vi "Turret_roller_module.vi"(0 "Reset":bool, 1 "Enable":bool, 2 "Ball Detected":bool, 3 "Ball too far":bool, 4 "Ball not far enough":bool, 5 "Lower Conveyor has Ball":bool, 6 "Shoot":bool) -> (14 "Turret Roller State":T1, 15 "T Roller Motor":dbl, 17 "Acquired Ball":bool, 18 "Accepting Balls":bool, 19 "Shot Ball":bool)   [LabVIEW 2012]
doc: "State machine for the roller buffer mounted on the turret between the tower conveyor and the flywheel."
uses:
  T_Roller module state.ctl
panel:
  in  "Shooting Timeout":u32=1000
  in  "Fast Speed":dbl=1.0
  in  "Slow Speed":dbl=0.3
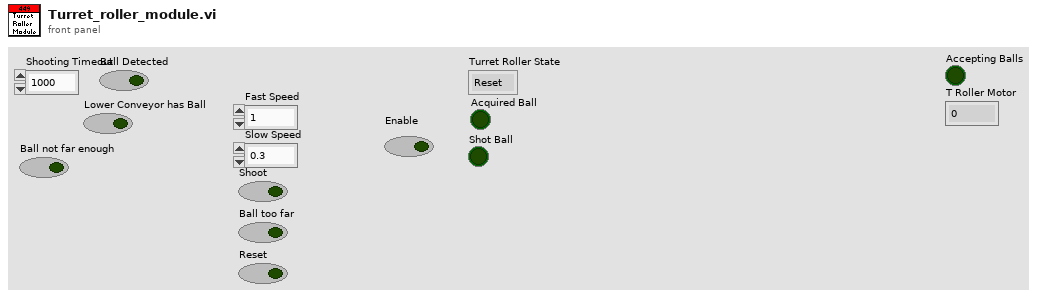
[diagram p1: front panel]
types:
  T1 = typedef "T_Roller module state.ctl" = enum16{"Reset", "Disabled", "Waiting for Ball", "Holding", "Ball not far enough", "Ball too far", "Firing"}
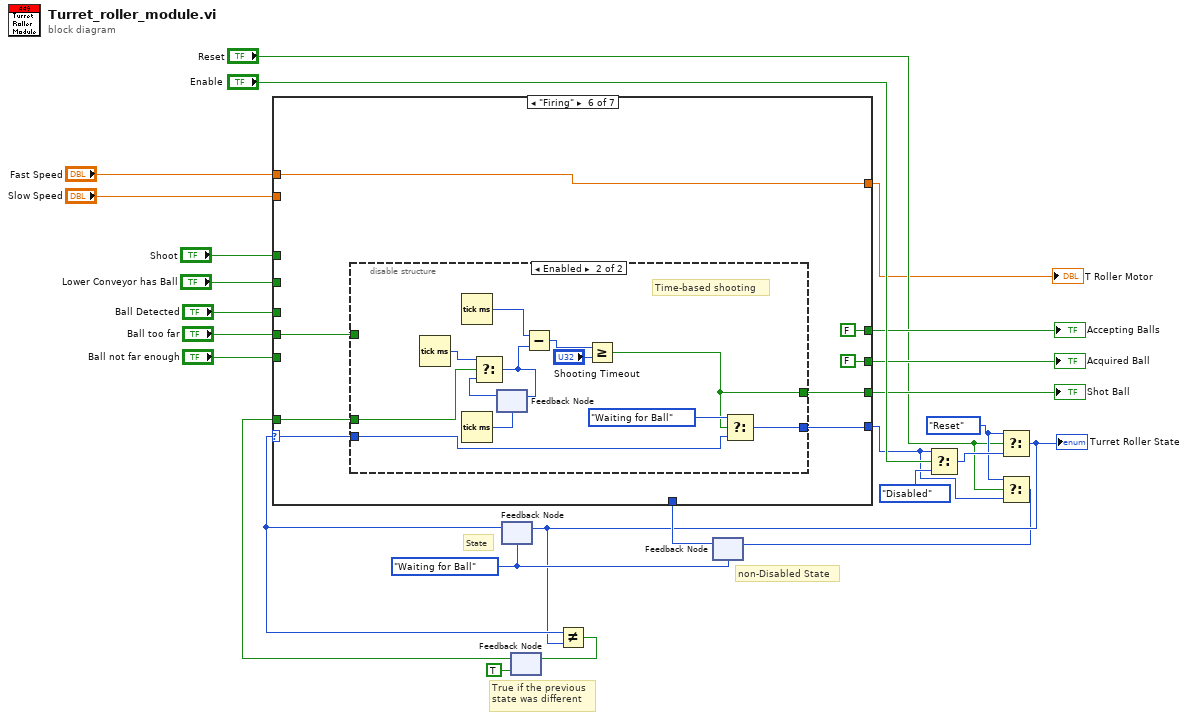
[diagram p0: block diagram]
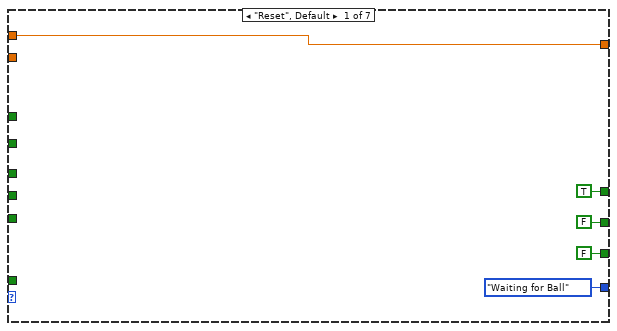
[diagram p2: hidden frame]
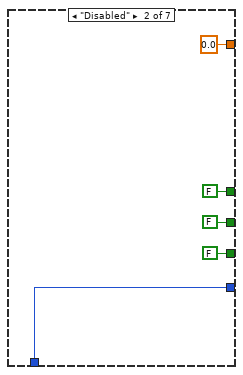
[diagram p3: hidden frame]
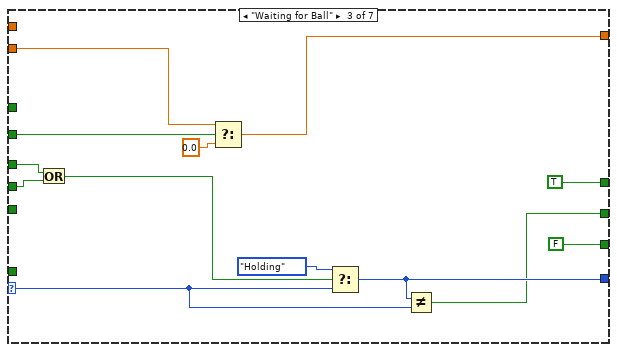
[diagram p4: hidden frame]
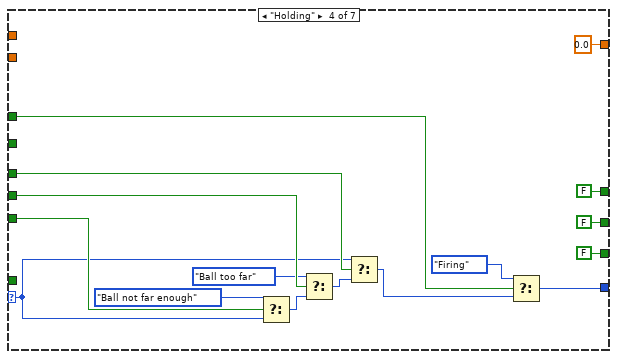
[diagram p5: hidden frame]
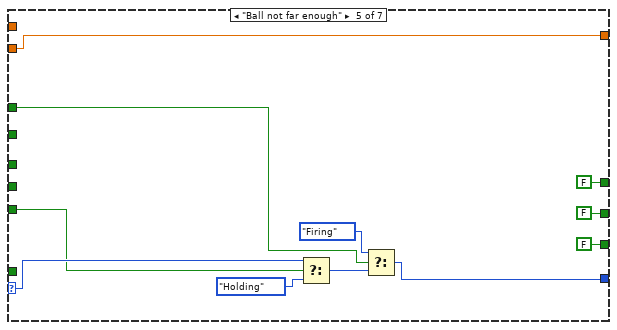
[diagram p6: hidden frame]
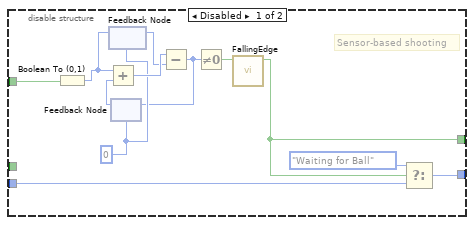
[diagram p7: hidden frame]
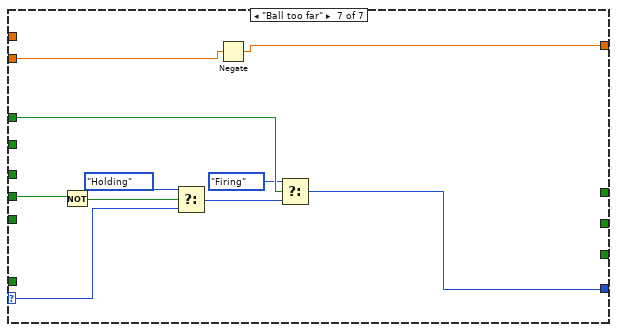
[diagram p8: hidden frame]
diagram:
  w13 = T_Roller_module_state."Reset" ("t")
  w7 = T_Roller_module_state."Waiting for Ball" ("Turret Roller Module State")
  # "True if the previous\nstate was different"
  # "State"
  # "non-Disabled State"
  n1 = feedback #1(w7) -> (w25:T1)
  n2 = feedback #2(TRUE) -> (w1:bool)
  n3 = feedback #3(w7) -> (w6:T1)
  n4 = case shown="\"Firing\"" w25 {
    selector: w25 -> [_ _ w39 w49 w75 w78 w113]
    tunnel: [w30 0.0 ("Fast Speed") w43 0.0 ("Slow Speed") w66 w83 w116] -> w10
    tunnel: "Fast Speed" -> [w30 _ _ _ _ w83 _]
    tunnel: "Slow Speed" -> [_ _ w44 _ w66 _ w117]
    tunnel: "Shoot" -> [_ _ _ w57 w67 _ w110]
    tunnel: "Ball Detected" -> [_ _ w38 w56 _ _ _]
    tunnel: "Ball too far" -> [_ _ w37 w54 _ w80 w115]
    tunnel: [T_Roller_module_state."Waiting for Ball" ("Turret Roller Module State") w31 w41 w60 w72 w79 w108] -> w11
    tunnel: [TRUE FALSE TRUE FALSE FALSE FALSE _] -> w16
    tunnel: [FALSE ("Ball Detected") FALSE ("Ball Detected") w40 FALSE ("Ball Detected") FALSE ("Ball Detected") FALSE ("Ball Detected") _] -> w15
    tunnel: [FALSE ("BooleanOut") FALSE ("BooleanOut") FALSE FALSE ("BooleanOut") FALSE w77 _] -> w14
    tunnel: w6 -> [_ w31 _ _ _ _ _]
    tunnel: "Lower Conveyor has Ball" -> [_ _ w46 _ _ _ _]
    tunnel: "Ball not far enough" -> [_ _ _ w51 w65 _ _]
    tunnel: w1 -> [_ _ _ _ _ w76 _]
    frame "Reset", Default {
    }
    frame "Disabled" {
    }
    frame "Waiting for Ball" {
      n5 = Or(x=w38, y=w37) -> (x .or. y?=w36:bool)
      n6 = Select(t=w44, s=w46, f=0.0) -> (s? t:f=w43:dbl)
      n7 = Select(t=T_Roller_module_state."Holding", s=w36, f=w39) -> (s? t:f=w41:T1)
      n8 = Not Equal?(x=w41, y=w39) -> (x != y?=w40:bool)
    }
    frame "Holding" {
      n9 = Select(t=T_Roller_module_state."Ball not far enough", s=w51, f=w49) -> (s? t:f=w52:T1)
      n10 = Select(t=T_Roller_module_state."Ball too far" ("f"), s=w54, f=w52) -> (s? t:f=w55:T1)
      n11 = Select(t=w49, s=w56, f=w55) -> (s? t:f=w59:T1)
      n12 = Select(t=T_Roller_module_state."Firing", s=w57, f=w59) -> (s? t:f=w60:T1)
    }
    frame "Ball not far enough" {
      n13 = Select(t=w75, s=w65, f=T_Roller_module_state."Holding") -> (s? t:f=w73:T1)
      n14 = Select(t=T_Roller_module_state."Firing", s=w67, f=w73) -> (s? t:f=w72:T1)
    }
    frame "Firing" {
      n15 = disable-structure shown="Enabled" {
        disable-tunnel: w80 -> [w95 _]
        disable-tunnel: [w87 w98] -> w79
        disable-tunnel: w78 -> [w86 w96]
        disable-tunnel: [w85 w97] -> w77
        disable-tunnel: w76 -> [_ w105]
        frame Disabled {
          w90 = i16 0
          # "Sensor-based shooting"
          n16 = Boolean To (0,1)(Boolean=w95) -> (0, 1=w91:i16)
          n17 = feedback #4(w90) -> (w92:i16)
          n18 = feedback-in #4(w91) -> ()
          n19 = feedback #5(w90) -> (w94:i16)
          n20 = Add(x=w91, y=w94) -> (x+y=w93:i16)
          n21 = Subtract(x=w93, y=w92) -> (x-y=w89:i16)
          n22 = feedback-in #5(w89) -> ()
          n23 = Not Equal To 0?(x=w89) -> (x != 0?=w88:bool)
          n24 = call "FallingEdge.vi"("BooleanIn"=w88) -> ("BooleanOut"=w85:bool)  [unwired: 10 in]
          n25 = Select(t=T_Roller_module_state."Waiting for Ball", s=w85, f=w86) -> (s? t:f=w87:T1)
        }
        frame Enabled {
          # "Time-based shooting"
          n26 = Tick Count (ms)() -> (millisecond timer value=w107:u32)
          n27 = Tick Count (ms)() -> (millisecond timer value=w102:u32)
          n28 = Tick Count (ms)() -> (millisecond timer value=w104:u32)
          n29 = feedback #6(w104) -> (w106:u32)
          n30 = Select(t=w107, s=w105, f=w106) -> (s? t:f=w103:u32)
          n31 = feedback-in #6(w103) -> ()
          n32 = Subtract(x=w102, y=w103) -> (x-y=w101:u32)
          n33 = Greater Or Equal?(x=w101, y="Shooting Timeout") -> (x >= y?=w97:bool)
          n34 = Select(t=T_Roller_module_state."Waiting for Ball" ("Turret Roller Module State"), s=w97, f=w96) -> (s? t:f=w98:T1)
        }
      }
    }
    frame "Ball too far" {
      n35 = Not(x=w115) -> (.not. x?=w114:bool)
      n36 = Select(t=T_Roller_module_state."Holding", s=w114, f=w113) -> (s? t:f=w111:T1)
      n37 = Negate(x=w117) -> (-x=w116:dbl)
      n38 = Select(t=T_Roller_module_state."Firing", s=w110, f=w111) -> (s? t:f=w108:T1)
    }
  }
  "T Roller Motor" <- w10
  "Accepting Balls" <- w16
  "Acquired Ball" <- w15
  "Shot Ball" <- w14
  n39 = Select(t=w11, s="Enable", f=T_Roller_module_state."Disabled" ("t")) -> (s? t:f=w22:T1)
  n40 = Select(t=w13, s="Reset", f=w22) -> (s? t:f=w5:T1)
  "Turret Roller State" <- w5
  n41 = feedback-in #1(w5) -> ()
  n42 = Not Equal?(x=w25, y=w5) -> (x != y?=w3:bool)
  n43 = feedback-in #2(w3) -> ()
  n44 = Select(t=w13, s="Reset", f=w11) -> (s? t:f=w4:T1)
  n45 = feedback-in #3(w4) -> ()
